vi "UTS PID.vi"() -> ()   [LabVIEW 2016]
panel:
  out "Waveform Susu":T1(graph)
  in  "Set Point Susu":dbl(slide) scale=0.0..100.0
  out "Error Aktual 3":dbl
  in  "Kp 3":dbl
  in  "Ki 3":dbl
  in  "Kd 3":dbl
  out "Waveform Gula":T1(graph)
  in  "Set Point Gula":dbl(slide) scale=0.0..100.0
  out "Error Aktual 2":dbl
  in  "Kp 2":dbl
  in  "Ki 2":dbl
  in  "Kd 2":dbl
  out "Waveform Kopi":T1(graph)
  out "Error Aktual":dbl
  in  "Kd":dbl
  in  "Ki":dbl
  in  "Kp":dbl
  in  "Set Point Kopi":dbl(slide) scale=0.0..100.0
  out "result 5":bool
  out "Kadar Susu 2":dbl
  out "Kadar Gula 2":dbl
  out "Kadar Kopi 2":dbl
  out "result 6":bool
  out "x > y?":bool
  out "y":bool
  out "Boolean 4":bool
  out "Boolean 3":bool
  out "Boolean 2":bool
  out "result 4":dbl
  out "result 3":dbl
  out "result 2":dbl
  out "concatenated string 3":string
  out "concatenated string 2":string
  out "concatenated string":string
  out "x*y 3":dbl
  out "x*y 2":dbl
  out "x*y":dbl
  out "%Kadar Susu":dbl(slide) scale=0.0..100.0
  out "%Kadar Gula":dbl(slide) scale=0.0..100.0
  out "%Kadar Kopi":dbl(slide) scale=0.0..100.0
  out "result":bool
  out "% Katup Susu":dbl
  out "% Katup Gula":dbl
  out "% Katup Kopi":dbl
  in  "Control Susu":dbl(slide) scale=0.0..100.0
  in  "Control Gula":dbl(slide) scale=0.0..100.0
  out "Susu":dbl(slide) scale=0.0..100.0
  out "Gula":dbl(slide) scale=0.0..100.0
  in  "stop":bool
  in  "Control Kopi":dbl(slide) scale=0.0..100.0
  in  "Control Output":dbl(slide) scale=0.0..100.0
  out "Time":dbl
  out "Output":dbl(slide) scale=0.0..100.0
  out "Kopi":dbl(slide) scale=0.0..100.0
  # "SIMULASI MESIN PENCAMPUR KOPI DENGAN MENGGUNAKAN PID"
  # "KONTROL GULA"
  # "KONTROL KOPI"
  # "KONTROL SUSU"
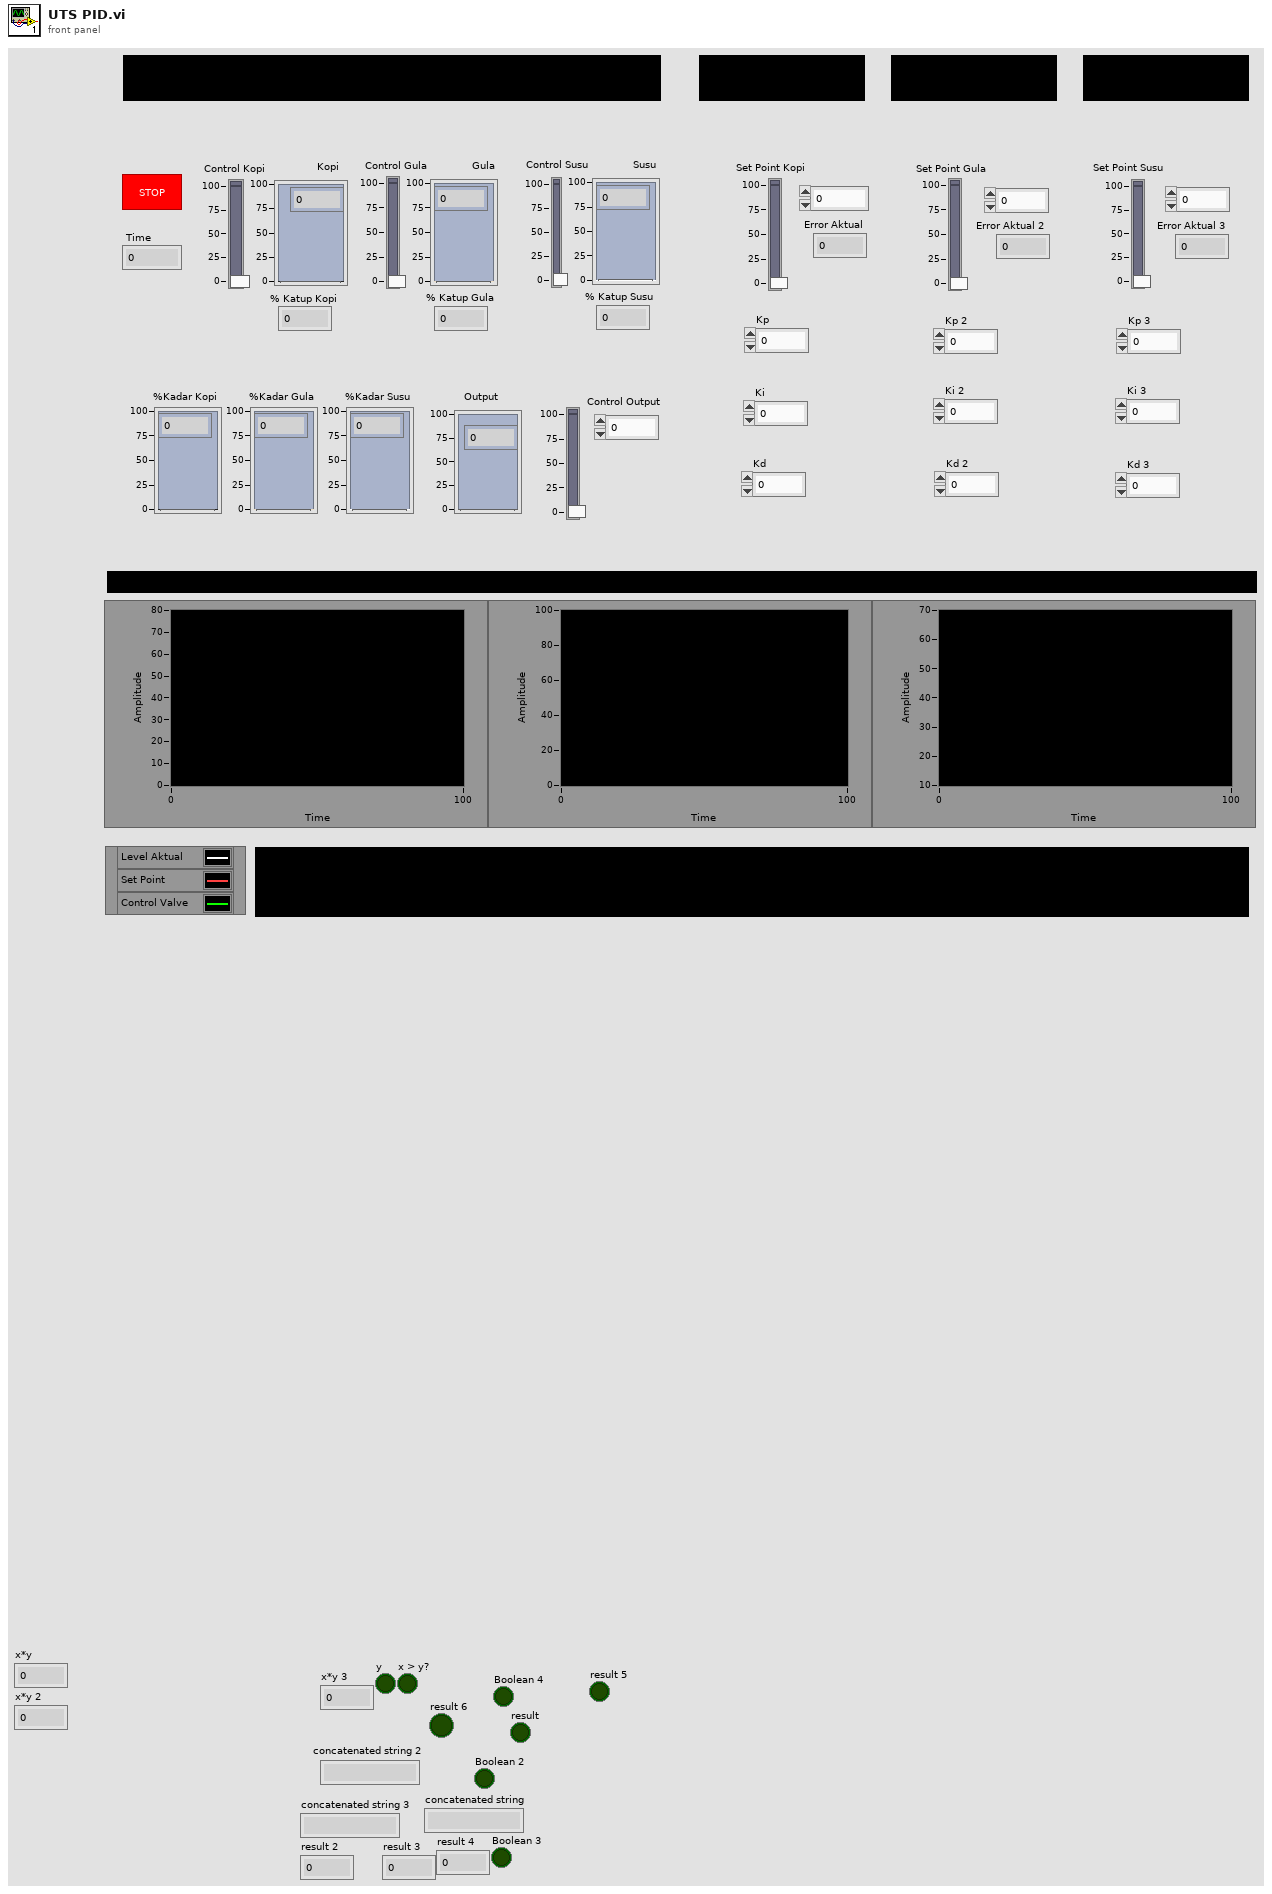
[diagram p1: front panel]
types:
  T1 = cluster{"Control Kopi":dbl, "Set Point Kopi":dbl, "%Kadar Kopi":dbl}
  T2 = cluster{"Kadar Kopi 2":dbl, "Set Point Kopi":dbl, "Control Kopi":dbl}
  T3 = cluster{"Kadar Susu 2":dbl, "Set Point Susu":dbl, " Control Susu":dbl}
  T4 = cluster{"Kadar Gula 2":dbl, "Set Point Gula":dbl, " Control Gula":dbl}
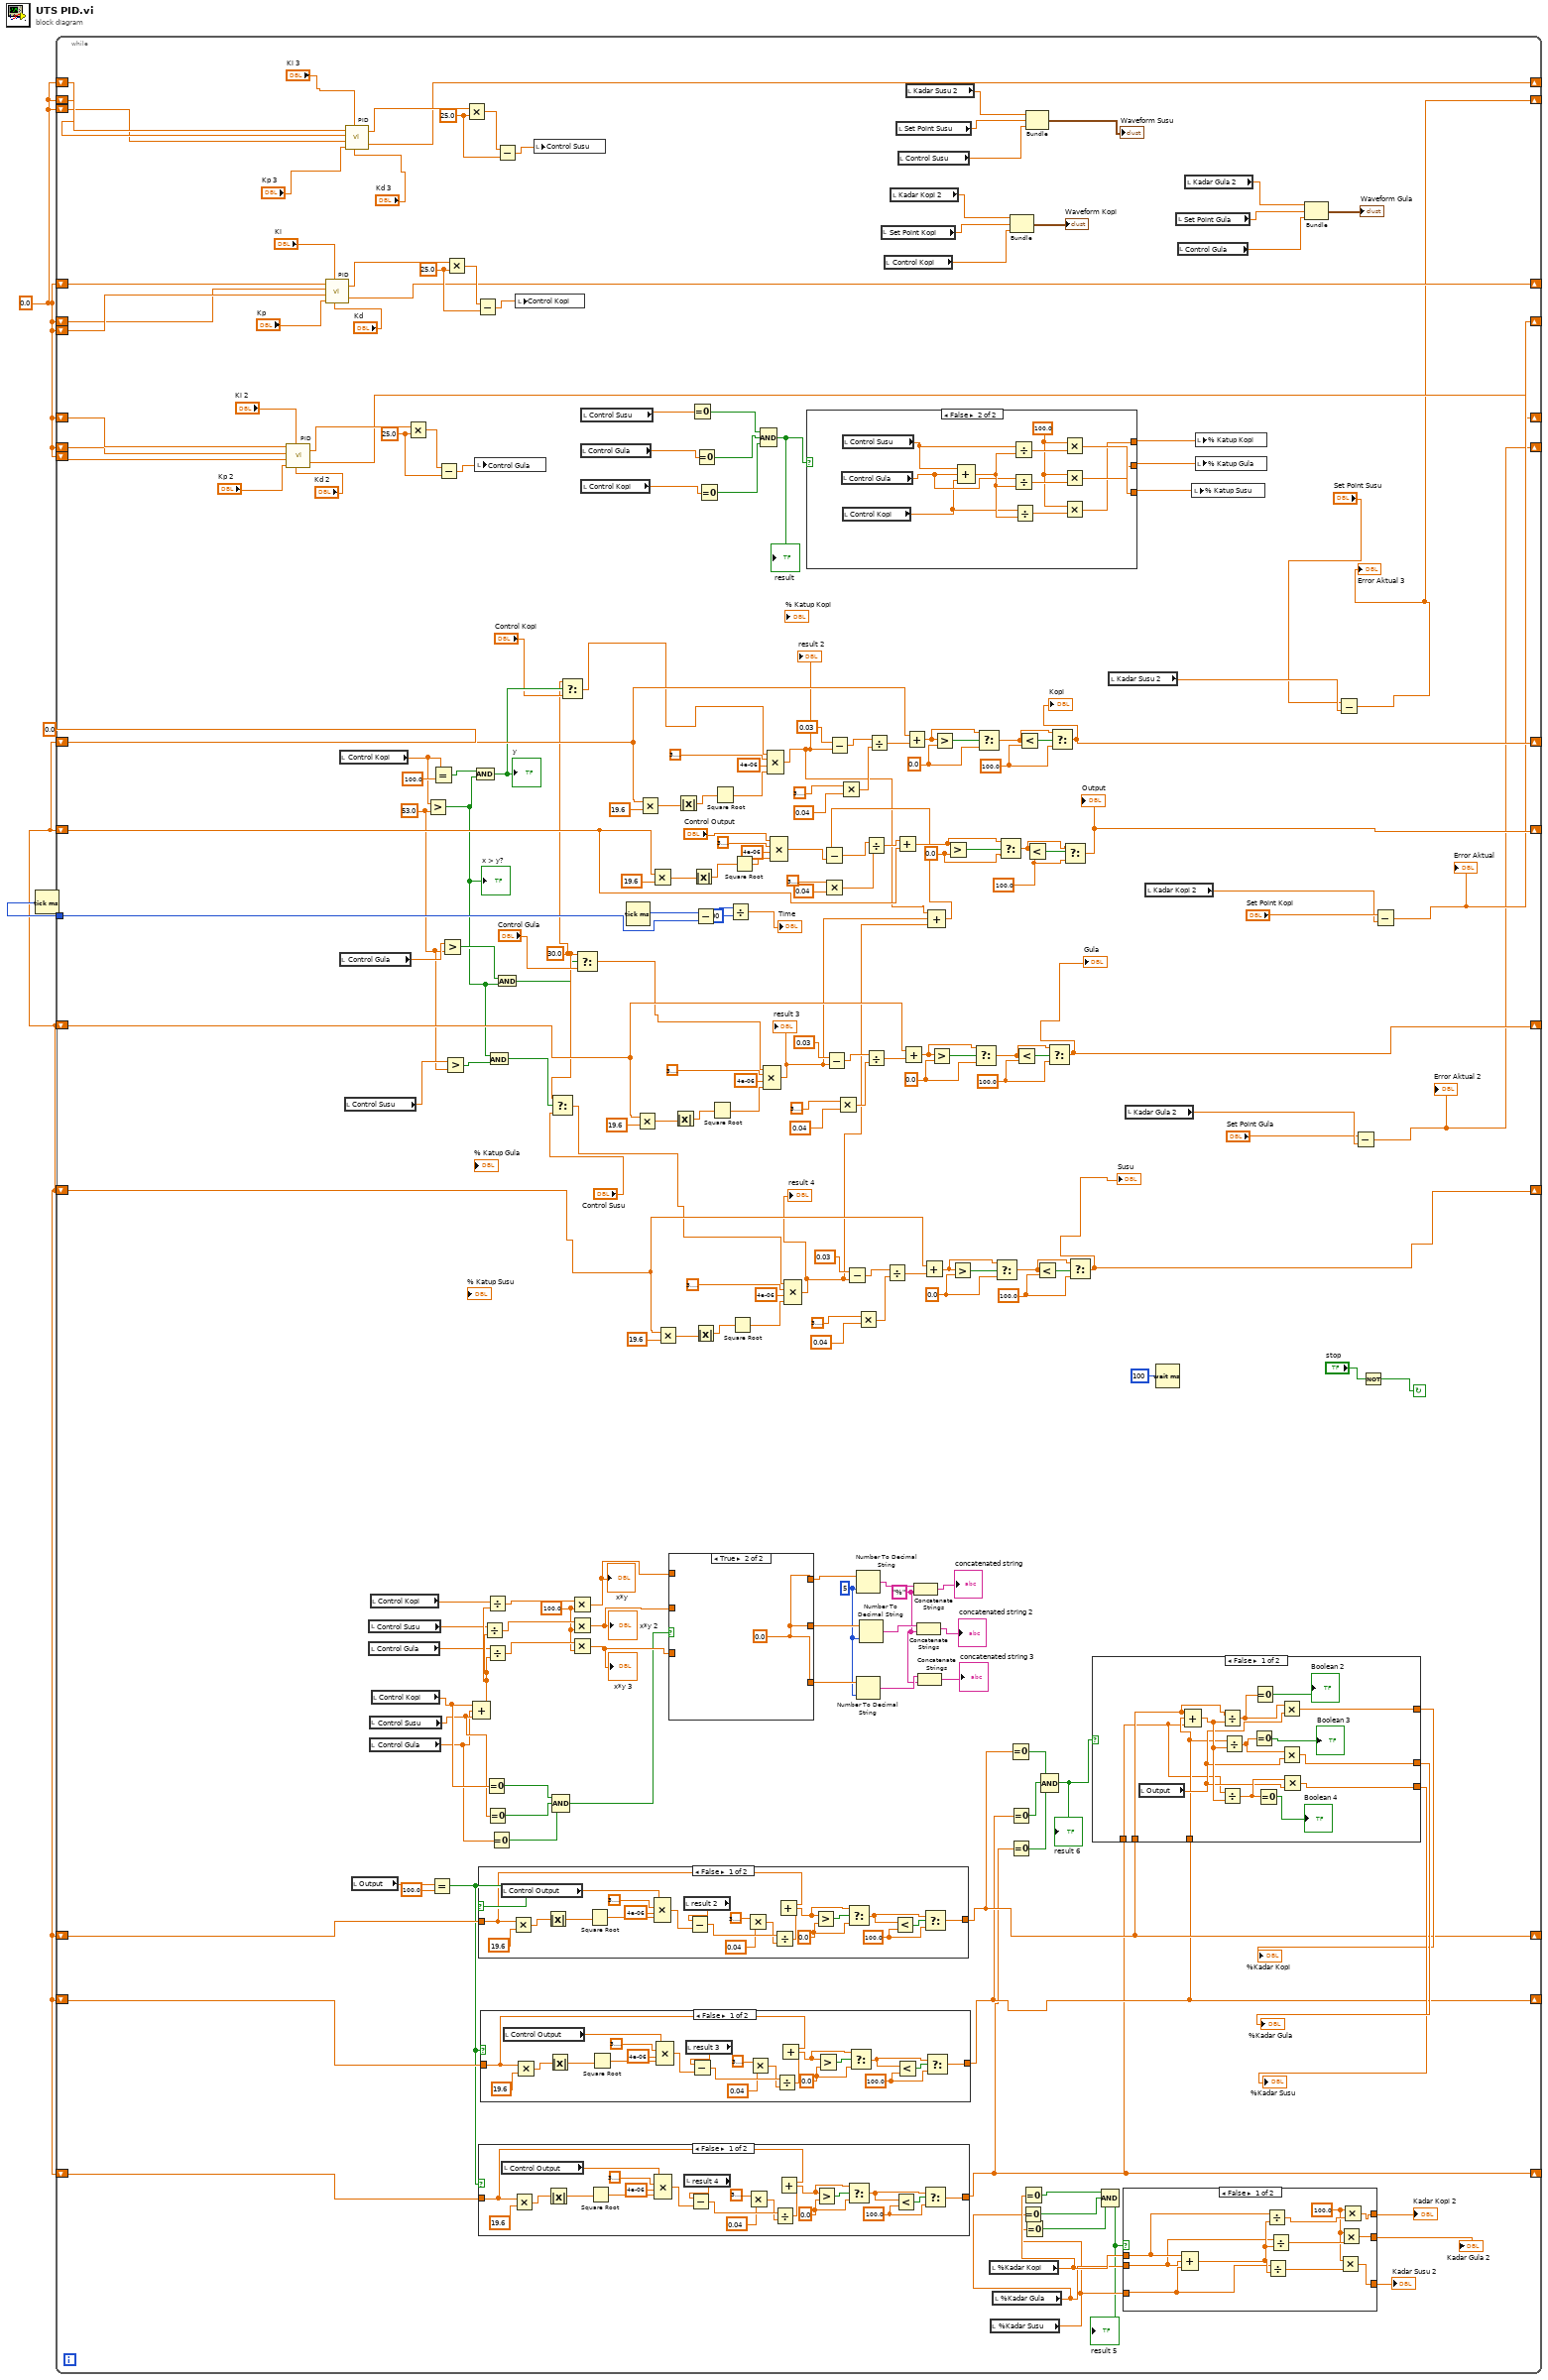
[diagram p0: block diagram]
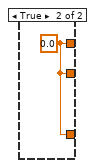
[diagram p2: hidden frame]
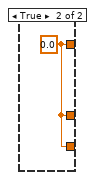
[diagram p3: hidden frame]
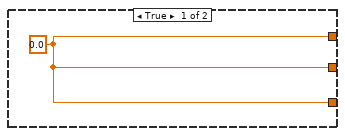
[diagram p8: hidden frame]
diagram:
  w1 = 0.0
  w2 = 0.0 ("y")
  n1 = Tick Count (ms)() -> (millisecond timer value=w3:u32)
  n2 = while {
    shift-right: [w141] -> _
    shift-left: w2 -> [w219]
    shift-right: [w46] -> _
    shift-left: w2 -> [w191]
    tunnel: w3 -> [w201]
    shift-right: [w48] -> _
    shift-left: w2 -> [w170]
    shift-right: [w47] -> _
    shift-left: w2 -> [w150]
    shift-right: [w73] -> _
    shift-left: w2 -> [w108]
    shift-right: [w72] -> _
    shift-left: w2 -> [w107]
    shift-right: [w71] -> _
    shift-left: w2 -> [w106]
    shift-right: [w50] -> _
    shift-left: w1 -> [w60]
    shift-right: [w45] -> _
    shift-left: w1 -> [w58]
    shift-left: w1 -> [w59]
    shift-right: [w29] -> _
    shift-left: w1 -> [w31]
    shift-right: [w26] -> _
    shift-left: w1 -> [w30]
    shift-left: w1 -> [w32]
    shift-right: [w11] -> _
    shift-left: w1 -> [w17]
    shift-right: [w8] -> _
    shift-left: w1 -> [w16]
    shift-left: w1 -> [w15]
    stop <- w195 continue-if-true
    w20 = 25.0 ("y")
    w38 = 25.0 ("y")
    w52 = 25.0 ("y")
    w88 = 53.0 ("y")
    w94 = 30.0 ("t")
    w119 = "%" ("string")
    w121 = i16 5 ("width (-)")
    w132 = 100.0 ("y")
    w155 = 100.0 ("y")
    w157 = 0.0 ("f")
    w175 = 100.0 ("y")
    w177 = 0.0 ("f")
    w202 = 100.0 ("y")
    w206 = 0.0 ("y")
    w221 = 100.0 ("y")
    w223 = 0.0 ("f")
    n3 = call "PID.vi"("Kd"="Kd 2", "Ki"="Ki 2", "Kp"="Kp 2", "error(t-2)"=w32, "error (t-1)"=w30, "error total(t-1)"=w31) -> ("Error Total (t)"=w29:dbl, "Sinyal Kontrol"=w36:dbl)
    n4 = call "PID.vi"("Kd"="Kd", "Ki"="Ki", "Kp"="Kp", "error(t-2)"=w59, "error (t-1)"=w58, "error total(t-1)"=w60) -> ("Error Total (t)"=w50:dbl, "Sinyal Kontrol"=w54:dbl)
    n5 = local read "Control Kopi"() -> (w92:dbl)
    n6 = local read "Control Gula"() -> (w89:dbl)
    n7 = local read "Control Susu"() -> (w90:dbl)
    n8 = call "PID.vi"("Kd"="Kd 3", "Ki"="Ki 3", "Kp"="Kp 3", "error(t-2)"=w15, "error (t-1)"=w16, "error total(t-1)"=w17) -> ("Error Total (t)"=w11:dbl, "Sinyal Kontrol"=w18:dbl)
    n9 = local read "Output"() -> (w110:dbl)
    n10 = local read "Control Susu"() -> (w137:dbl)
    n11 = local read "Control Gula"() -> (w136:dbl)
    n12 = local read "Control Susu"() -> (w116:dbl)
    n13 = local read "Control Gula"() -> (w115:dbl)
    n14 = local read "Control Kopi"() -> (w138:dbl)
    n15 = local read "Control Kopi"() -> (w117:dbl)
    n16 = Multiply(x=w36, y=w38) -> (x*y=w37:dbl)
    n17 = Greater?(x=w92, y=w88) -> (0:w87:bool)
    "x > y?" <- w87
    n18 = Equal?(x=w110, y=100.0) -> (x = y?=w105:bool)
    n19 = Equal?(x=w92, y=100.0) -> (x = y?=w102:bool)
    n20 = Subtract(x=w37, y=w38) -> (x-y=w39:dbl)
    n21 = Greater?(x=w89, y=w88) -> (0:w91:bool)
    n22 = Greater?(x=w90, y=w88) -> (0:w86:bool)
    n23 = Multiply(x=w54, y=w52) -> (x*y=w53:dbl)
    n24 = Multiply(x=w18, y=w20) -> (x*y=w19:dbl)
    n25 = Compound Arithmetic op=ADD(w117, w115, w116) -> (w139:dbl)
    n26 = And(x=w102, y=w87) -> (x .and. y?=w101:bool)
    "y" <- w101
    n27 = local write "Control Gula"(w39) -> ()
    n28 = Subtract(x=w53, y=w52) -> (x-y=w51:dbl)
    n29 = case shown="False" w105 {
      tunnel: w108 -> [w314 w330]
      tunnel: [w309 w330] -> w73
      frame False {
        w310 = 100.0 ("y")
        w313 = 0.0 ("y")
        n30 = local read "Control Output"() -> (w323:dbl)
        n31 = Multiply(x=w314, y=19.6) -> (x*y=w328:dbl)
        n32 = Absolute Value(x=w328) -> (abs(x)=w327:dbl)
        n33 = Square Root(x=w327) -> (sqrt(x)=w326:dbl)
        n34 = Compound Arithmetic op=MULTIPLY(w323, 3.141592653589793, 4e-06 ("value"), w326) -> (w322:dbl)
        n35 = local read "result 2"() -> (w321:dbl)
        n36 = Subtract(x=w321, y=w322) -> (x-y=w320:dbl)
        n37 = Multiply(x=3.141592653589793, y=0.04 ("value")) -> (x*y=w319:dbl)
        n38 = Divide(x=w320, y=w319) -> (x/y=w316:dbl)
        n39 = Add(x=w314, y=w316) -> (x+y=w308:dbl)
        n40 = Greater?(x=w308, y=w313) -> (0:w315:bool)
        n41 = Select(t=w308, s=w315, f=w313) -> (s? t:f=w311:dbl)
        n42 = Less?(x=w311, y=w310) -> (x < y?=w312:bool)
        n43 = Select(t=w311, s=w312, f=w310) -> (s? t:f=w309:dbl)
      }
      frame True {
      }
    }
    n44 = case shown="False" w105 {
      tunnel: w106 -> [w268 w284]
      tunnel: [w263 w284] -> w71
      frame False {
        w264 = 100.0 ("y")
        w267 = 0.0 ("y")
        n45 = local read "Control Output"() -> (w277:dbl)
        n46 = Multiply(x=w268, y=19.6) -> (x*y=w282:dbl)
        n47 = Absolute Value(x=w282) -> (abs(x)=w281:dbl)
        n48 = Square Root(x=w281) -> (sqrt(x)=w280:dbl)
        n49 = Compound Arithmetic op=MULTIPLY(w277, 3.141592653589793, 4e-06 ("value"), w280) -> (w276:dbl)
        n50 = local read "result 4"() -> (w275:dbl)
        n51 = Subtract(x=w275, y=w276) -> (x-y=w274:dbl)
        n52 = Multiply(x=3.141592653589793, y=0.04 ("value")) -> (x*y=w273:dbl)
        n53 = Divide(x=w274, y=w273) -> (x/y=w270:dbl)
        n54 = Add(x=w268, y=w270) -> (x+y=w262:dbl)
        n55 = Greater?(x=w262, y=w267) -> (0:w269:bool)
        n56 = Select(t=w262, s=w269, f=w267) -> (s? t:f=w265:dbl)
        n57 = Less?(x=w265, y=w264) -> (x < y?=w266:bool)
        n58 = Select(t=w265, s=w266, f=w264) -> (s? t:f=w263:dbl)
      }
      frame True {
      }
    }
    n59 = case shown="False" w105 {
      tunnel: w107 -> [w291 w307]
      tunnel: [w286 w307] -> w72
      frame False {
        w287 = 100.0 ("y")
        w290 = 0.0 ("y")
        n60 = local read "Control Output"() -> (w300:dbl)
        n61 = Multiply(x=w291, y=19.6) -> (x*y=w305:dbl)
        n62 = Absolute Value(x=w305) -> (abs(x)=w304:dbl)
        n63 = Square Root(x=w304) -> (sqrt(x)=w303:dbl)
        n64 = Compound Arithmetic op=MULTIPLY(w300, 3.141592653589793, 4e-06 ("value"), w303) -> (w299:dbl)
        n65 = local read "result 3"() -> (w298:dbl)
        n66 = Subtract(x=w298, y=w299) -> (x-y=w297:dbl)
        n67 = Multiply(x=3.141592653589793, y=0.04 ("value")) -> (x*y=w296:dbl)
        n68 = Divide(x=w297, y=w296) -> (x/y=w293:dbl)
        n69 = Add(x=w291, y=w293) -> (x+y=w285:dbl)
        n70 = Greater?(x=w285, y=w290) -> (0:w292:bool)
        n71 = Select(t=w285, s=w292, f=w290) -> (s? t:f=w288:dbl)
        n72 = Less?(x=w288, y=w287) -> (x < y?=w289:bool)
        n73 = Select(t=w288, s=w289, f=w287) -> (s? t:f=w286:dbl)
      }
      frame True {
      }
    }
    n74 = Divide(x=w137, y=w139) -> (x/y=w134:dbl)
    n75 = Equal To 0?(x=w117) -> (x = 0?=w114:bool)
    n76 = Divide(x=w138, y=w139) -> (x/y=w135:dbl)
    n77 = Divide(x=w136, y=w139) -> (x/y=w133:dbl)
    n78 = Equal To 0?(x=w116) -> (x = 0?=w113:bool)
    n79 = And(x=w87, y=w86) -> (x .and. y?=w85:bool)
    n80 = Equal To 0?(x=w115) -> (x = 0?=w112:bool)
    n81 = Subtract(x=w19, y=w20) -> (x-y=w21:dbl)
    n82 = And(x=w91, y=w87) -> (x .and. y?=w84:bool)
    n83 = local write "Control Kopi"(w51) -> ()
    n84 = local write "Control Susu"(w21) -> ()
    n85 = Select(t=w94, s=w85, f="Control Susu") -> (s? t:f=w97:dbl)
    n86 = Compound Arithmetic op=AND(w114, w113, w112) -> (w111:bool)
    n87 = Select(t=w94, s=w101, f="Control Kopi") -> (s? t:f=w100:dbl)
    n88 = Multiply(x=w135, y=w132) -> (x*y=w131:dbl)
    "x*y" <- w131
    n89 = Multiply(x=w134, y=w132) -> (x*y=w130:dbl)
    "x*y 2" <- w130
    n90 = Multiply(x=w133, y=w132) -> (x*y=w129:dbl)
    "x*y 3" <- w129
    n91 = Select(t=w94, s=w84, f="Control Gula") -> (s? t:f=w98:dbl)
    n92 = local read "Control Gula"() -> (w147:dbl)
    n93 = local read "Control Susu"() -> (w148:dbl)
    n94 = local read "Control Kopi"() -> (w146:dbl)
    n95 = Tick Count (ms)() -> (millisecond timer value=w200:u32)
    n96 = Multiply(x=w170, y=19.6) -> (x*y=w187:dbl)
    n97 = Multiply(x=w219, y=19.6) -> (x*y=w233:dbl)
    n98 = Multiply(x=w191, y=19.6) -> (x*y=w218:dbl)
    n99 = Multiply(x=w150, y=19.6) -> (x*y=w167:dbl)
    n100 = case shown="True" w111 {
      tunnel: w131 -> [w333 _]
      tunnel: w130 -> [w332 _]
      tunnel: w129 -> [w331 _]
      tunnel: [w333 w334] -> w128
      tunnel: [w332 w334] -> w127
      tunnel: [w331 w334] -> w122
      frame False {
      }
      frame True {
        w334 = 0.0 ("y")
      }
    }
    n101 = Absolute Value(x=w187) -> (abs(x)=w186:dbl)
    n102 = Absolute Value(x=w233) -> (abs(x)=w232:dbl)
    n103 = Equal To 0?(x=w148) -> (x = 0?=w145:bool)
    n104 = Absolute Value(x=w218) -> (abs(x)=w217:dbl)
    n105 = Subtract(x=w200, y=w201) -> (x-y=w199:u32)
    n106 = Absolute Value(x=w167) -> (abs(x)=w166:dbl)
    n107 = Equal To 0?(x=w147) -> (x = 0?=w144:bool)
    n108 = Equal To 0?(x=w146) -> (x = 0?=w143:bool)
    n109 = Square Root(x=w186) -> (sqrt(x)=w185:dbl)
    n110 = Square Root(x=w232) -> (sqrt(x)=w231:dbl)
    n111 = Divide(x=w199, y=u32 1000) -> (x/y=→"Time":dbl)
    n112 = Square Root(x=w166) -> (sqrt(x)=w165:dbl)
    n113 = Square Root(x=w217) -> (sqrt(x)=w216:dbl)
    n114 = Compound Arithmetic op=AND(w145, w144, w143) -> (w142:bool)
    "result" <- w142
    n115 = Compound Arithmetic op=MULTIPLY(w98, 3.141592653589793, 4e-06 ("value"), w185) -> (w104:dbl)
    "result 3" <- w104
    n116 = Compound Arithmetic op=MULTIPLY(w100, 3.141592653589793, 4e-06 ("value"), w231) -> (w140:dbl)
    "result 2" <- w140
    n117 = Compound Arithmetic op=MULTIPLY("Control Output", 3.141592653589793, 4e-06 ("value"), w216) -> (w212:dbl)
    n118 = Compound Arithmetic op=MULTIPLY(w97, 3.141592653589793, 4e-06 ("value"), w165) -> (w103:dbl)
    "result 4" <- w103
    n119 = case shown="False" w142 {
      tunnel: [w335 w336] -> w83
      tunnel: [w335 w337] -> w82
      tunnel: [w335 w338] -> w81
      frame True {
        w335 = 0.0 ("%kopi")
      }
      frame False {
        w339 = 100.0
        n120 = local read "Control Gula"() -> (w344:dbl)
        n121 = local read "Control Susu"() -> (w345:dbl)
        n122 = local read "Control Kopi"() -> (w343:dbl)
        n123 = Compound Arithmetic op=ADD(w345, w344, w343) -> (w346:dbl)
        n124 = Divide(x=w345, y=w346) -> (x/y=w342:dbl)
        n125 = Divide(x=w344, y=w346) -> (x/y=w341:dbl)
        n126 = Divide(x=w343, y=w346) -> (x/y=w340:dbl)
        n127 = Multiply(x=w339, y=w342) -> (x*y=w338:dbl)
        n128 = Multiply(x=w339, y=w341) -> (x*y=w337:dbl)
        n129 = Multiply(x=w339, y=w340) -> (x*y=w336:dbl)
      }
    }
    n130 = Multiply(x=3.141592653589793, y=0.04) -> (x*y=w210:dbl)
    n131 = Subtract(x=0.03, y=w104) -> (x-y=w183:dbl)
    n132 = Subtract(x=0.03, y=w140) -> (x-y=w229:dbl)
    n133 = Multiply(x=3.141592653589793, y=0.04) -> (x*y=w182:dbl)
    n134 = Multiply(x=3.141592653589793, y=0.04) -> (x*y=w228:dbl)
    n135 = Subtract(x=0.03, y=w103) -> (x-y=w163:dbl)
    n136 = Number To Decimal String(number=w122, width (-)=w121) -> (decimal integer string=w120:string)
    n137 = Multiply(x=3.141592653589793, y=0.04) -> (x*y=w162:dbl)
    n138 = Number To Decimal String(number=w128, width (-)=w121) -> (decimal integer string=w126:string)
    n139 = Number To Decimal String(number=w127, width (-)=w121) -> (decimal integer string=w125:string)
    n140 = Divide(x=w183, y=w182) -> (x/y=w181:dbl)
    n141 = Divide(x=w229, y=w228) -> (x/y=w227:dbl)
    n142 = local read "Set Point Kopi"() -> (w42:dbl)
    n143 = local read "Control Kopi"() -> (w41:dbl)
    n144 = Divide(x=w163, y=w162) -> (x/y=w161:dbl)
    n145 = local read "Kadar Kopi 2"() -> (w43:dbl)
    n146 = local read "Set Point Susu"() -> (w6:dbl)
    n147 = local read "Control Susu"() -> (w5:dbl)
    n148 = Add(x=w170, y=w181) -> (x+y=w178:dbl)
    n149 = Add(x=w219, y=w227) -> (x+y=w224:dbl)
    n150 = local read "Kadar Susu 2"() -> (w7:dbl)
    n151 = Concatenate Strings(w126, w119) -> (→"concatenated string":string)
    n152 = Concatenate Strings(w125, w119) -> (→"concatenated string 2":string)
    n153 = Concatenate Strings(w120, w119) -> (→"concatenated string 3":string)
    n154 = Add(x=w150, y=w161) -> (x+y=w158:dbl)
    n155 = Compound Arithmetic op=ADD(w140, w104, w103) -> (w169:dbl)
    n156 = Subtract(x=w169, y=w212) -> (x-y=w211:dbl)
    n157 = Divide(x=w211, y=w210) -> (x/y=w192:dbl)
    n158 = Add(x=w192, y=w191) -> (x+y=w205:dbl)
    n159 = Greater?(x=w178, y=w177) -> (0:w179:bool)
    n160 = Greater?(x=w224, y=w223) -> (0:w225:bool)
    n161 = Greater?(x=w205, y=w206) -> (0:w207:bool)
    n162 = Greater?(x=w158, y=w157) -> (0:w159:bool)
    n163 = Select(t=w178, s=w179, f=w177) -> (s? t:f=w174:dbl)
    n164 = Select(t=w224, s=w225, f=w223) -> (s? t:f=w220:dbl)
    n165 = local read "%Kadar Kopi"() -> (w67:dbl)
    n166 = local read "%Kadar Susu"() -> (w65:dbl)
    n167 = local read "%Kadar Gula"() -> (w66:dbl)
    n168 = Select(t=w158, s=w159, f=w157) -> (s? t:f=w154:dbl)
    n169 = Select(t=w205, s=w207, f=w206) -> (s? t:f=w203:dbl)
    n170 = Equal To 0?(x=w73) -> (x = 0?=w80:bool)
    n171 = Equal To 0?(x=w72) -> (x = 0?=w79:bool)
    n172 = Equal To 0?(x=w71) -> (x = 0?=w78:bool)
    n173 = Bundle("Kadar Kopi 2"=w43, "Set Point Kopi"=w42, "Control Kopi"=w41) -> (→"Waveform Kopi":T2)  [unwired: 1 in]
    n174 = Less?(x=w174, y=w175) -> (x < y?=w176:bool)
    n175 = Less?(x=w220, y=w221) -> (x < y?=w222:bool)
    n176 = Equal To 0?(x=w66) -> (x = 0?=w63:bool)
    n177 = Equal To 0?(x=w67) -> (x = 0?=w64:bool)
    n178 = Equal To 0?(x=w65) -> (x = 0?=w62:bool)
    n179 = Bundle("Kadar Susu 2"=w7, "Set Point Susu"=w6, "Control Susu"=w5) -> (→"Waveform Susu":T3)  [unwired: 1 in]
    n180 = Less?(x=w203, y=w202) -> (x < y?=w204:bool)
    n181 = Less?(x=w154, y=w155) -> (x < y?=w156:bool)
    n182 = Compound Arithmetic op=AND(w80, w79, w78) -> (w77:bool)
    "result 6" <- w77
    n183 = Select(t=w174, s=w176, f=w175) -> (s? t:f=w48:dbl)
    "Gula" <- w48
    n184 = Select(t=w220, s=w222, f=w221) -> (s? t:f=w141:dbl)
    "Kopi" <- w141
    n185 = Select(t=w203, s=w204, f=w202) -> (s? t:f=w46:dbl)
    "Output" <- w46
    n186 = Select(t=w154, s=w156, f=w155) -> (s? t:f=w47:dbl)
    "Susu" <- w47
    n187 = case shown="False" w77 {
      tunnel: [w250 w261] -> w74
      tunnel: [w255 w261] -> w76
      tunnel: [w254 w261] -> w75
      tunnel: w73 -> [w249 _]
      tunnel: w72 -> [w248 _]
      tunnel: w71 -> [w247 _]
      frame False {
        n188 = local read "Output"() -> (w251:dbl)
        n189 = Compound Arithmetic op=ADD(w249, w248, w247) -> (w260:dbl)
        n190 = Divide(x=w249, y=w260) -> (x/y=w256:dbl)
        n191 = Divide(x=w247, y=w260) -> (x/y=w252:dbl)
        n192 = Divide(x=w248, y=w260) -> (x/y=w253:dbl)
        n193 = Equal To 0?(x=w253) -> (x = 0?=→"Boolean 3":bool)
        n194 = Equal To 0?(x=w256) -> (x = 0?=→"Boolean 2":bool)
        n195 = Equal To 0?(x=w252) -> (x = 0?=→"Boolean 4":bool)
        n196 = Multiply(x=w256, y=w251) -> (x*y=w250:dbl)
        n197 = Multiply(x=w253, y=w251) -> (x*y=w255:dbl)
        n198 = Multiply(x=w252, y=w251) -> (x*y=w254:dbl)
      }
      frame True {
        w261 = 0.0
      }
    }
    "%Kadar Kopi" <- w74
    "%Kadar Gula" <- w76
    "%Kadar Susu" <- w75
    n199 = Compound Arithmetic op=AND(w64, w63, w62) -> (w61:bool)
    "result 5" <- w61
    n200 = local read "Kadar Susu 2"() -> (w10:dbl)
    n201 = case shown="False" w61 {
      tunnel: w67 -> [w240 _]
      tunnel: w66 -> [w239 _]
      tunnel: w65 -> [w238 _]
      tunnel: [w237 w246] -> w70
      tunnel: [w236 w246] -> w69
      tunnel: [w235 w246] -> w68
      frame False {
        w241 = 100.0 ("x")
        n202 = Compound Arithmetic op=ADD(w240, w239, w238) -> (w245:dbl)
        n203 = Divide(x=w240, y=w245) -> (x/y=w244:dbl)
        n204 = Divide(x=w238, y=w245) -> (x/y=w242:dbl)
        n205 = Divide(x=w239, y=w245) -> (x/y=w243:dbl)
        n206 = Multiply(x=w241, y=w242) -> (x*y=w235:dbl)
        n207 = Multiply(x=w241, y=w243) -> (x*y=w236:dbl)
        n208 = Multiply(x=w241, y=w244) -> (x*y=w237:dbl)
      }
      frame True {
        w246 = 0.0
      }
    }
    "Kadar Kopi 2" <- w70
    "Kadar Gula 2" <- w69
    "Kadar Susu 2" <- w68
    n209 = local read "Kadar Gula 2"() -> (w28:dbl)
    n210 = local read "Kadar Kopi 2"() -> (w44:dbl)
    n211 = Wait (ms)(milliseconds to wait=u32 100) -> ()  [unwired: 1 out]
    n212 = local read "Set Point Gula"() -> (w23:dbl)
    n213 = local read "Control Gula"() -> (w24:dbl)
    n214 = local read "Kadar Gula 2"() -> (w22:dbl)
    n215 = local write "% Katup Susu"(w81) -> ()
    n216 = local write "% Katup Kopi"(w83) -> ()
    n217 = local write "% Katup Gula"(w82) -> ()
    n218 = Bundle("Kadar Gula 2"=w22, "Set Point Gula"=w23, "Control Gula"=w24) -> (→"Waveform Gula":T4)  [unwired: 1 in]
    n219 = Subtract(x="Set Point Susu", y=w10) -> (x-y=w8:dbl)
    "Error Aktual 3" <- w8
    n220 = Subtract(x="Set Point Gula", y=w28) -> (x-y=w26:dbl)
    "Error Aktual 2" <- w26
    n221 = Not(x="stop") -> (.not. x?=w195:bool)
    n222 = Subtract(x="Set Point Kopi", y=w44) -> (x-y=w45:dbl)
    "Error Aktual" <- w45
  }
